vi "Endpoint Connected.vi"(8 "error in":errorcluster, 10 "Endpoint":refnum<class "Message Enqueuer.lvclass">, 11 "Host MSS Test Actor in":refnum<class "Host MSS Test Actor.lvclass">) -> (0 "error out":errorcluster, 3 "Host MSS Test Actor out":refnum<class "Host MSS Test Actor.lvclass">)   [LabVIEW 2023, in "Host MSS Test Actor.lvlib" / "Host MSS Test Actor.lvclass"]
doc: "Override this method to specify how the receiving actor responds to a Connected message from a nested endpoint actor."
uses:
  <vilib>/ActorFramework/Message Enqueuer/Message Enqueuer.lvclass
  Host MSS Test Actor.lvclass
  Host MSS Test Actor.lvclass/Host MSS Test Actor.ctl
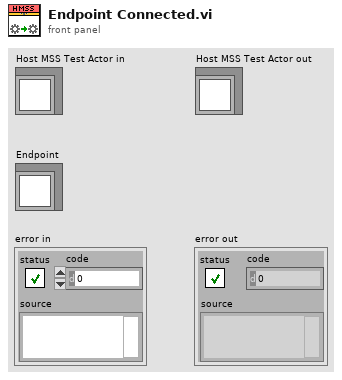
[diagram p1: front panel]
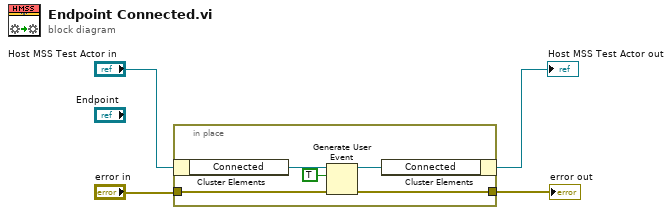
[diagram p0: block diagram]
diagram:
  n1 = in-place {
    in-place-border: "error in" -> [w7]
    in-place-border: [w6] -> w1
    n2 = in-place-cluster #1("Host MSS Test Actor in") -> ("Connected"=w9:refnum<user-event>)
    n3 = Generate User Event(user event=w9, event data cluster=TRUE ("event data"), error in=w7) -> (user event out=w8:refnum<user-event>, error out=w6:errorcluster)  [unwired: 1 in]
    n4 = in-place-cluster #1("Connected"=w8) -> (→"Host MSS Test Actor out":refnum<class "Host MSS Test Actor.lvclass">)
  }
  "error out" <- w1
